vi "WHH Equation.vi"(10 "h":dbl, 11 "t":dbl) -> (3 "WHH(x)":dbl format="%.19f")   [LabVIEW 2021]
uses:
  <vilib>/gmath/NI_Gmath.lvlib
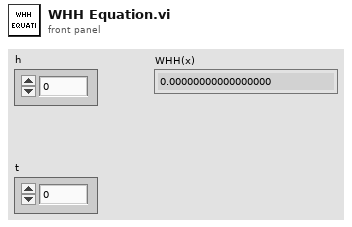
[diagram p1: front panel]
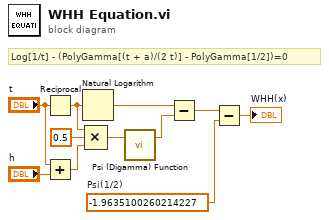
[diagram p0: block diagram]
diagram:
  w1 = -1.9635100260214227  # Psi(1/2)
  # "Log[1/t] - (PolyGamma[(t + a)/(2 t)] - PolyGamma[1/2])=0"
  n1 = Reciprocal(x="t") -> (1/x=w9:dbl)
  n2 = Add(x="t", y="h") -> (x+y=w10:dbl)
  n3 = Natural Logarithm(1:w9) -> (0:w5:dbl)
  n4 = Compound Arithmetic op=MULTIPLY(w9, 0.5, w10) -> (w6:dbl)
  n5 = call <vilib>:"Psi (Digamma) Function.vi"("x"=w6) -> ("y(x)"=w3:dbl)  [unwired: 2 in]
  n6 = Subtract(x=w5, y=w3) -> (x-y=w4:dbl)
  n7 = Subtract(x=w4, y=w1) -> (x-y=→"WHH(x)":dbl)
